vi "Set Destination Path.vi"(8 "error in (no error)":errorcluster, 9 "Destination path":path, 10 "Destination label":string, 11 "PPL in":refnum<class "NI_AB_API_PPL.lvclass">) -> (0 "error out":errorcluster, 3 "PPL out":refnum<class "NI_AB_API_PPL.lvclass">)   [LabVIEW 2020, in "NI_AB_API_PPL.lvclass"]
uses:
  <vilib>/AppBuilder/AB_API/PPL/NI_AB_API_PPL.lvclass
  <vilib>/AppBuilder/AB_API/Targetfile/NI_AB_API_Targetfile.lvclass
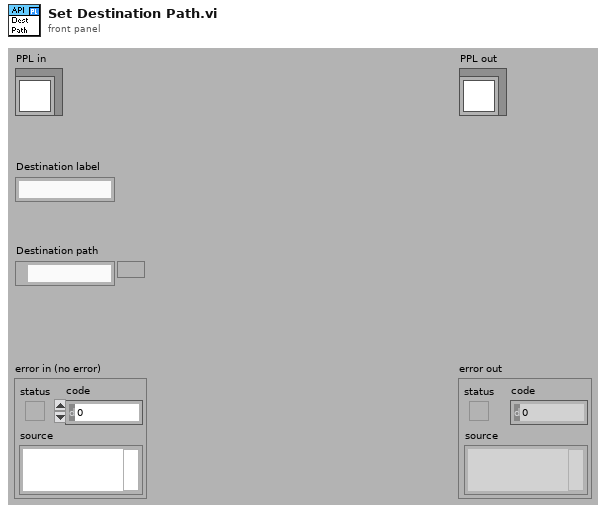
[diagram p1: front panel]
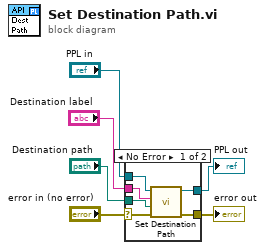
[diagram p0: block diagram]
diagram:
  n1 = case shown="No Error" "error in (no error)" {
    selector: "error in (no error)" -> [w9 w14]
    tunnel: [w10 w14] -> w2
    tunnel: [w11 w13] -> w1
    tunnel: "PPL in" -> [w12 w13]
    tunnel: "Destination label" -> [w7 _]
    tunnel: "Destination path" -> [w8 _]
    frame No Error {
      n2 = call-parent "Set Destination Path.vi"("error in (no error)"=w9, "Destination path"=w8, "Destination label"=w7, "Build in"=w12) -> ("error out"=w10:errorcluster, "Build out"=w11:refnum<class "NI_AB_API_PPL.lvclass">)  [unwired: 6 in]
    }
    frame Error {
    }
  }
  "error out" <- w2
  "PPL out" <- w1
